vi "test Configuration.vi"(8 "error in (no error)":errorcluster, 11 "BC Configuration in":refnum<class "BC Configuration.lvclass">) -> (0 "error out":errorcluster, 3 "BC Configuration out":refnum<class "BC Configuration.lvclass">)   [LabVIEW 2016, in "BC Configuration.lvclass"]
uses:
  BC Configuration.lvclass
  D:/SVN/Products/SLSC/Multichannel 1553 Module/Software/Source Code/Driver (Windows)/Unit Tests/1553 Test/1553 Test.lvclass
  PPLs/FPGA Interface.lvlibp/FPGA Interface/FPGA Interface.lvclass
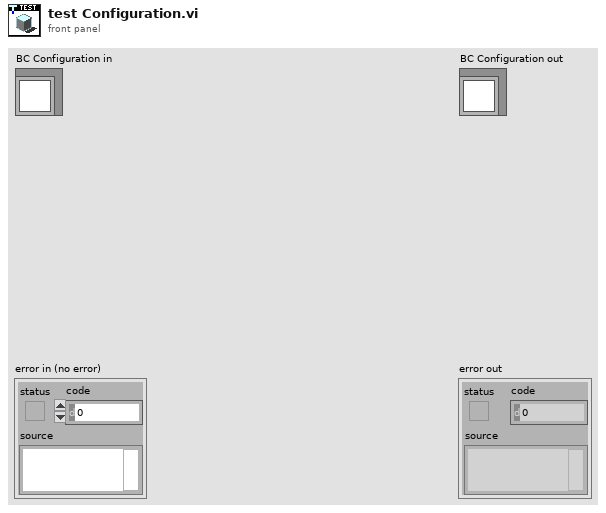
[diagram p1: front panel]
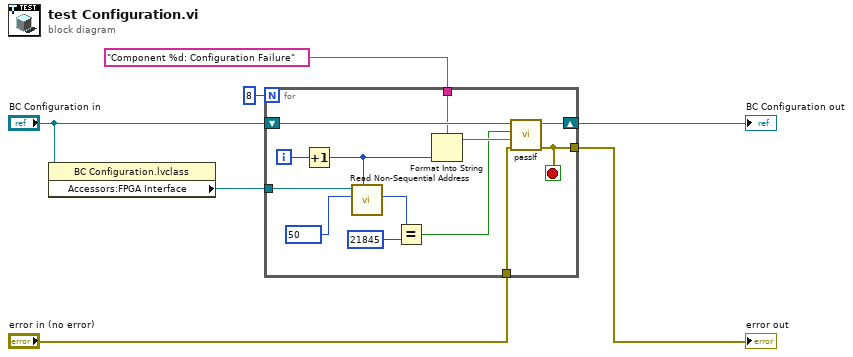
[diagram p0: block diagram]
diagram:
  n1 = property class="BC Configuration.lvclass"(reference="BC Configuration in") -> ("Accessors:FPGA Interface"=w7:refnum<class "FPGA Interface.lvclass">)  [unwired: 1 in, 2 out]
  n2 = for {
    N: 8 -> [_]
    tunnel: w7 -> [w20]
    shift-right: [w15] -> w5
    shift-left: "BC Configuration in" -> [w16]
    tunnel: "Component %d: Configuration Failure" ("custom report message (\"\")") -> [w14]
    tunnel: "error in (no error)" -> [w9]
    tunnel: [w8] -> w2
    i -> [w19]
    stop <- w8 stop-if-true
    n3 = Increment(x=w19) -> (x+1=w13:i32)
    n4 = call-dynamic "Read Non-Sequential Address.vi"("Target IC (1-8)"=w13, "Address"=u16 50, "FPGA Interface in"=w20) -> ("Data"=w11:u16)  [unwired: 7 in, 1 out]
    n5 = Equal?(x=w11, y=u16 21845) -> (x = y?=w10:bool)
    n6 = Format Into String(format string=w14, w13) -> (resulting string=w12:string)  [unwired: 2 in, 1 out]
    n7 = call-dynamic "passIf.vi"("error in (no error)"=w9, "message (\"\")"=w12, "pass"=w10, "TestCase in"=w16) -> ("error out"=w8:errorcluster, "TestCase out"=w15:refnum<class "BC Configuration.lvclass">)  [unwired: 6 in]
  }
  "error out" <- w2
  "BC Configuration out" <- w5
